vi "Get Firmware Pogram Interface Index.vi"(8 "Error In":errorcluster, 11 "Firmware Program Interface":string) -> (0 "Error Out":errorcluster, 3 "Interface Index":i32)   [LabVIEW 2013, in "LVH-LINX.lvlib"]
doc: "Get Firmware Program Interface enum index from string name."
uses:
  <vilib>/LabVIEW Hacker/LINX/LVH-LINX.lvlib
panel:
  in  "Firmware Program Interface":enum16{"N/A", "Serial / USB", "USB", "TCP"}(ring)
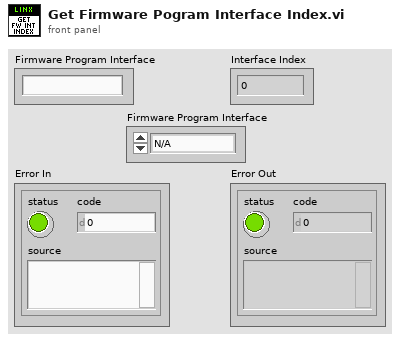
[diagram p1: front panel]
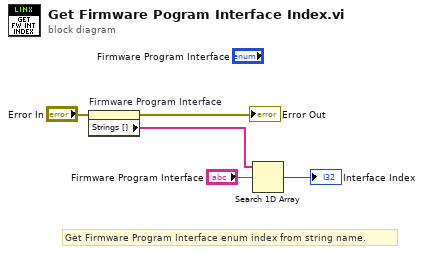
[diagram p0: block diagram]
diagram:
  # "Get Firmware Program Interface enum index from string name."
  n1 = property on="Firmware Program Interface" class="Enum (strict)"(error in="Error In") -> (error out=→"Error Out":errorcluster, "Strings []"=w5:string[])  [unwired: 1 in, 1 out]
  n2 = Search 1D Array(1D array=w5, element="Firmware Program Interface") -> (index of element=→"Interface Index":i32)  [unwired: 1 in]
